vi "Servomotores.vi"() -> ()   [LabVIEW 2024]
uses:
  <vilib>/Instr/_visa.llb/VISA Configure Serial Port (Instr).vi
panel:
  in  "VISA resource name":refnum<visa-resource-name>
  in  "Detener":bool
  out "Ángulo":string
  in  "Dial":dbl(knob) scale=0.0..180.0
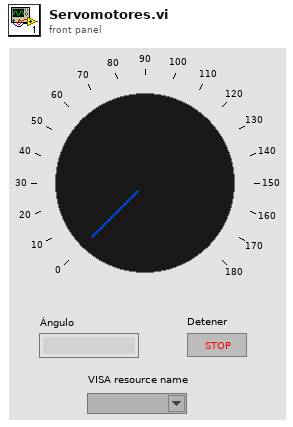
[diagram p1: front panel]
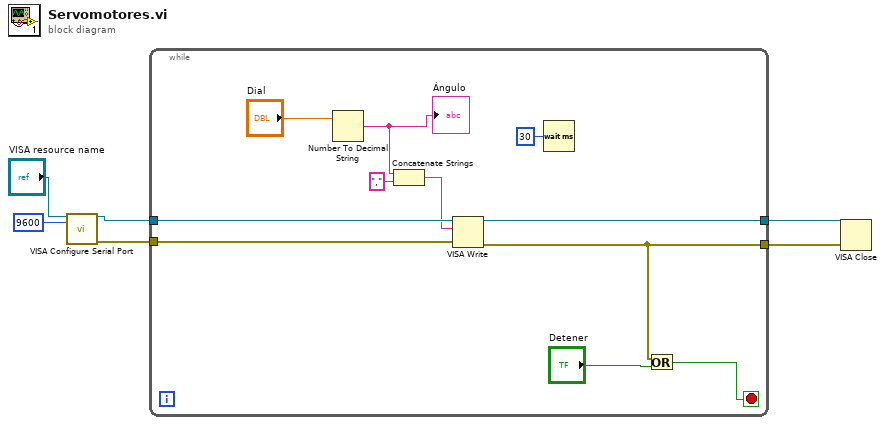
[diagram p0: block diagram]
diagram:
  n1 = call-poly "VISA Configure Serial Port"("VISA resource name"="VISA resource name", "baud rate (9600)"=u32 9600) -> ("VISA resource name out"=w2:refnum<visa-resource-name>, "error out"=w4:errorcluster)  [unwired: 12 in]
  n2 = while {
    tunnel: w4 -> [w15]
    tunnel: [w14] -> w3
    tunnel: w2 -> [w13]
    tunnel: [w12] -> w1
    stop <- w17 stop-if-true
    n3 = Number To Decimal String(number="Dial") -> (decimal integer string=w10:string)  [unwired: 1 in]
    "Ángulo" <- w10
    n4 = Concatenate Strings(w10, "," ("string")) -> (w9:string)
    n5 = VISA Write(VISA resource name=w13, write buffer=w9, error in (no error)=w15) -> (VISA resource name out=w12:refnum<visa-resource-name>, error out=w14:errorcluster)  [unwired: 1 out]
    n6 = Wait (ms)(milliseconds to wait=u32 30) -> ()  [unwired: 1 out]
    n7 = Or(x=w14, y="Detener") -> (x .or. y?=w17:bool)
  }
  n8 = VISA Close(VISA resource name=w1, error in (no error)=w3) -> ()  [unwired: 1 out]
